vi "H5Tget_member_name.vi"(6 "error in (no error)":errorcluster, 8 "Index":u32, 9 "HDF5 Compount Type Ref":T1) -> (0 "error out":errorcluster, 2 "name":string, 3 "HDF5 Ref out":T1)   [LabVIEW 2017]
doc: "Retrieves the name of a compound or enumeration datatype member."
uses:
  <vilib>/UPVI/lvhdf5/library.llb/HDF5 Ref.ctl
  <vilib>/UPVI/lvhdf5/h5helper.dll
panel:
  # "LVHDF5 Toolkit\nCopyright (c) 2005-2013 by Jason D. Sommerville\nCopyright (c) 2014 by UPVI, LLC.\n\nThis use and distribution of this file is governed by the terms found in \nLICENSE.txt distributed with this toolkit and installed at\n <user.lib>\\_lvhdf5\\LICENSE.txt"
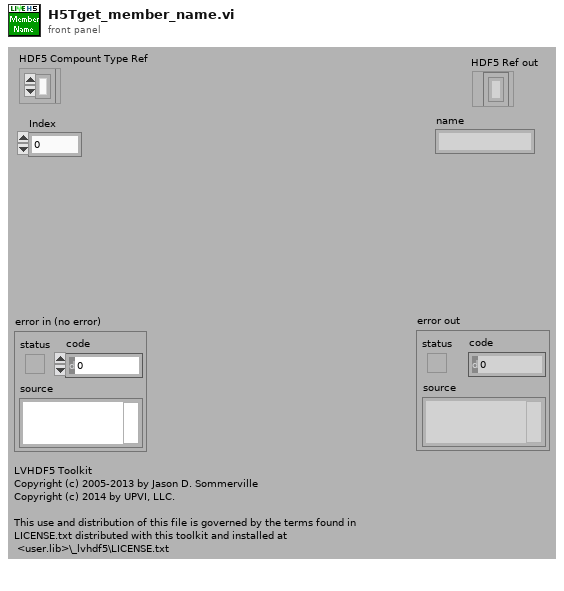
[diagram p1: front panel]
types:
  T1 = typedef "HDF5 Ref.ctl" = refnum<k1>
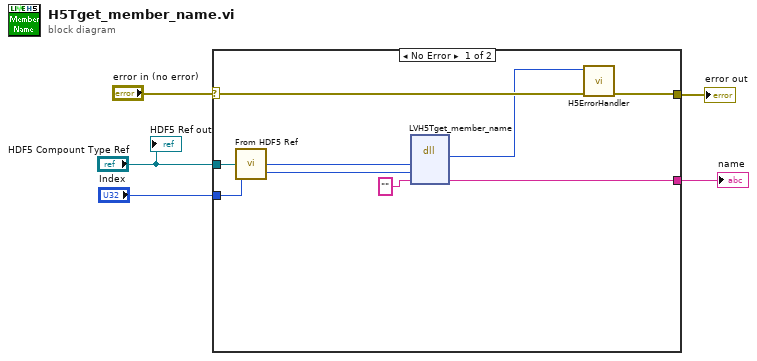
[diagram p0: block diagram]
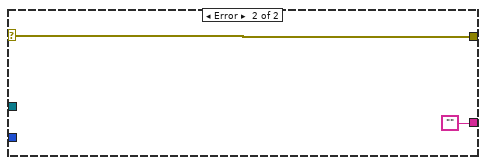
[diagram p2: hidden frame]
diagram:
  n1 = case shown="No Error" "error in (no error)" {
    selector: "error in (no error)" -> [w13 w15]
    tunnel: [w12 w15] -> w4
    tunnel: "HDF5 Compount Type Ref" -> [w10 _]
    tunnel: "Index" -> [w8 _]
    tunnel: [w6 ""] -> w1
    frame No Error {
      n2 = call <vilib>:"From HDF5 Ref.vi"("HDF5 Ref"=w10) -> ("I32"=w9:i32)
      n3 = dll-call lib="C:/Program Files/National Instruments/LabVIEW 2017/vi.lib/UPVI/lvhdf5/h5helper.dll" fn="LVH5Tget_member_name"("type_id"=w9, "index"=w8, "name"="") -> ("return type"=w11:i32, "name"=w6:string)  [unwired: 5 in, 2 out]
      n4 = call <vilib>:"H5ErrorHandler.vi"("error in (no error)"=w13, "herr_t"=w11) -> ("error out"=w12:errorcluster)  [unwired: 3 in, 4 out]
    }
    frame Error {
    }
  }
  "error out" <- w4
  "name" <- w1
  "HDF5 Ref out" <- "HDF5 Compount Type Ref"
